vi "Get Status.vi"(6 "timeout (ms)":i32=5000, 8 "error in":errorcluster, 11 "gRPC ID":T10) -> (0 "error out":errorcluster, 2 "Node Status":T1 {"Monitor Doubles"."4" format="%#_9g"; "Monitor Doubles"."3" format="%#_9g"; "Monitor Doubles"."2" format="%#_9g"; "Monitor Doubles"."1" format="%#_9g"}, 3 "gRPC ID out":T10)   [LabVIEW 2021, in "CIFCorePluginWrapper.lvlib"]
uses:
  CIFCorePluginWrapper.lvlib
  <vilib>/gRPC/LabVIEW gRPC Library/Shared/grpcId.ctl
  Common/Typedef/gRPC Reported Plugin Status.ctl
  Common/Typedef/Plugin State.ctl
  Common/Typedef/Timing Statistics.ctl
  Common/Typedef/Timing Stats Base.ctl
  Common/Typedef/FIFO Statistics.ctl
  Common/Typedef/Simple Error.ctl
  Common/Typedef/Monitor Doubles.ctl
  Common/Typedef/Monitor U64.ctl
  Common/Typedef/Monitor I64.ctl
  CIFCorePlugin_client/CIFCorePlugin_client.lvlib
  Common/CIFCoreCommon.lvlib
  <vilib>/gRPC/LabVIEW gRPC Library/grpc-lvsupport-release.lvlib
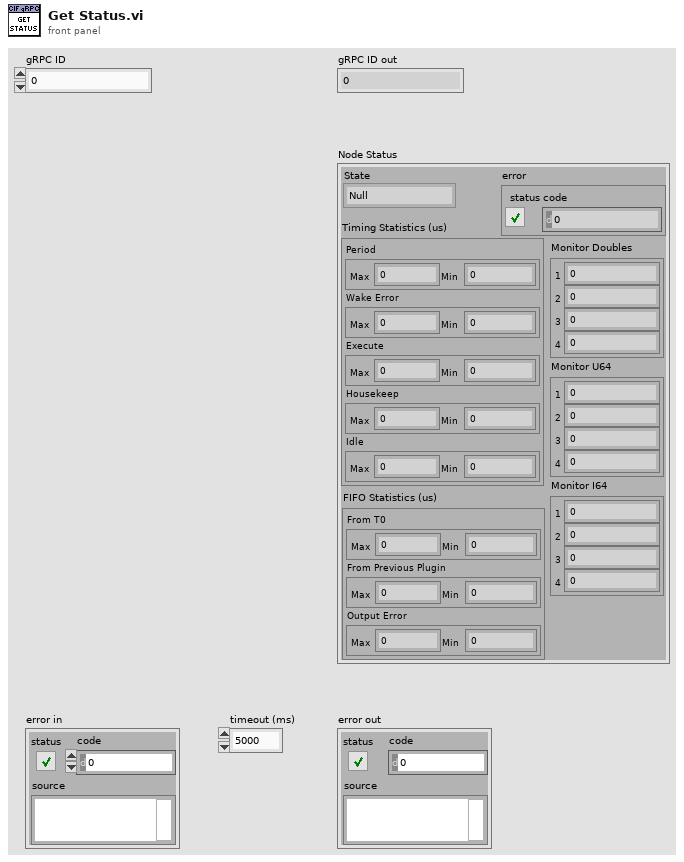
[diagram p1: front panel]
types:
  T1 = typedef "CIFCoreCommon.lvlib/gRPC Reported Plugin Status.ctl" = cluster{"State":T2, "Timing Statistics (us)":T3, "FIFO Statistics (us)":T5, "error":T6, "Monitor Doubles":T7, "Monitor U64":T8, "Monitor I64":T9}
  T2 = typedef "CIFCoreCommon.lvlib/Plugin State.ctl" = enum32{"Null", "Creating", "Listening", "Running", "CleaningUp", "Destroying"}
  T3 = typedef "CIFCoreCommon.lvlib/Timing Statistics.ctl" = cluster{"Period":T4, "Wake Error":T4, "Execute":T4, "Housekeep":T4, "Idle":T4}
  T4 = typedef "CIFCoreCommon.lvlib/Timing Stats Base.ctl" = cluster{"Max":i32, "Min":i32}
  T5 = typedef "CIFCoreCommon.lvlib/FIFO Statistics.ctl" = cluster{"From T0":T4, "From Previous Plugin":T4, "Output Error":T4}
  T6 = typedef "CIFCoreCommon.lvlib/Simple Error.ctl" = cluster{"status":bool, "code":i32}
  T7 = typedef "CIFCoreCommon.lvlib/Monitor Doubles.ctl" = cluster{"1":dbl, "2":dbl, "3":dbl, "4":dbl}
  T8 = typedef "CIFCoreCommon.lvlib/Monitor U64.ctl" = cluster{"1":u64, "2":u64, "3":u64, "4":u64}
  T9 = typedef "CIFCoreCommon.lvlib/Monitor I64.ctl" = cluster{"1":i64, "2":i64, "3":i64, "4":i64}
  T10 = typedef "grpc-lvsupport-release.lvlib/grpcId.ctl" = u64
  T11 = typedef "CIFCorePlugin_client.lvlib/cif_plugincore_StatusData.ctl" = cluster{"state":T12, "timing_statistics":T13, "fifo_statistics":T15, "error":T16, "monitor_doubles":T17, "monitor_u64s":T18, "monitor_i64s":T19}
  T12 = typedef "CIFCorePlugin_client.lvlib/cif_plugincore_StatusData_State.ctl" = enum32{"NULL", "CREATING", "LISTENING", "RUNNING", "CLEANINGUP", "DESTROYING"}
  T13 = typedef "CIFCorePlugin_client.lvlib/cif_plugincore_TimingStatistics.ctl" = cluster{"period":T14, "wake_error":T14, "execute":T14, "housekeep":T14, "idle":T14}
  T14 = typedef "CIFCorePlugin_client.lvlib/cif_plugincore_TimingStatsBasic.ctl" = cluster{"max":i32, "min":i32}
  T15 = typedef "CIFCorePlugin_client.lvlib/cif_plugincore_FifoStatistics.ctl" = cluster{"from_t0":T14, "from_previous_plugin":T14, "output_error":T14}
  T16 = typedef "CIFCorePlugin_client.lvlib/cif_plugincore_Error.ctl" = cluster{"status":bool, "code":i32}
  T17 = typedef "CIFCorePlugin_client.lvlib/cif_plugincore_MonitorDoubles.ctl" = cluster{"double_1":dbl, "double_2":dbl, "double_3":dbl, "double_4":dbl}
  T18 = typedef "CIFCorePlugin_client.lvlib/cif_plugincore_MonitorU64.ctl" = cluster{"u64_1":u64, "u64_2":u64, "u64_3":u64, "u64_4":u64}
  T19 = typedef "CIFCorePlugin_client.lvlib/cif_plugincore_MonitorI64.ctl" = cluster{"i64_1":i64, "i64_2":i64, "i64_3":i64, "i64_4":i64}
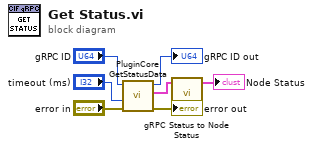
[diagram p0: block diagram]
diagram:
  n1 = call "PluginCore GetStatusData.vi"("error in"="error in", "timeout (ms)"="timeout (ms)", "gRPC ID"="gRPC ID") -> ("error out"=→"error out":errorcluster, "Response Data"=w2:T11, "gRPC ID out"=→"gRPC ID out":T10)  [unwired: 6 in]
  n2 = call "gRPC Status to Node Status.vi"("gRPC Status"=w2) -> ("Node Status"=→"Node Status":T1)  [unwired: 3 in]
